vi "MKS 946 Close.vi"(8 "error in (no error)":errorcluster, 11 "VISA resource name (IN)":refnum<visa-resource-name>) -> (0 "error out":errorcluster)   [LabVIEW 2013]
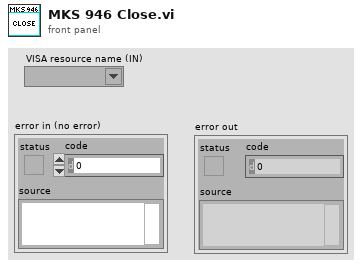
[diagram p1: front panel]
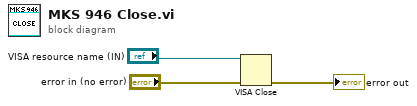
[diagram p0: block diagram]
diagram:
  n1 = VISA Close(VISA resource name="VISA resource name (IN)", error in (no error)="error in (no error)") -> (error out=→"error out":errorcluster)
